vi "DSF.Engine.Runtime.Get ID.vi"(8 "error in (no error)":errorcluster, 11 "Runtime in":refnum<class "DSF.Engine.Runtime.lvclass">) -> (0 "error out":errorcluster, 2 "id":i32, 3 "Runtime out":refnum<class "DSF.Engine.Runtime.lvclass">)   [LabVIEW 2016, in "DSF.Engine.lvlib" / "DSF.Engine.Runtime.lvclass"]
uses:
  DSF.Engine.Runtime.lvclass
  DSF.Engine.Runtime.lvclass/DSF.Engine.Runtime.ctl
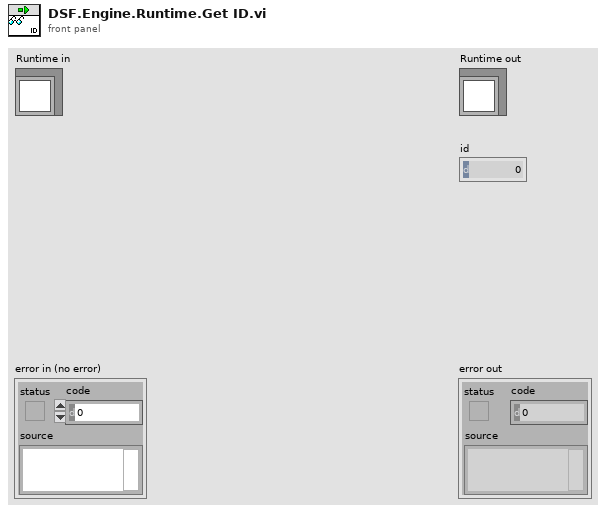
[diagram p1: front panel]
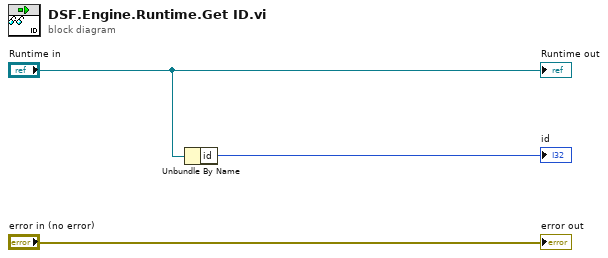
[diagram p0: block diagram]
diagram:
  n1 = Unbundle By Name("Runtime in") -> ("id"=→"id":i32)
  "error out" <- "error in (no error)"
  "Runtime out" <- "Runtime in"
